vi "Cursor-Controlled Subarray.vi"(0 "cursor graph":refnum<vi>, 1 "X":dbl[](array[numeric]), 2 "Y":dbl[](array[numeric])) -> (3 "X subset":dbl[](array[numeric]), 4 "Y subset":dbl[](array[numeric]), 5 "cursor avg":dbl, 6 "cursor diff":dbl)   [LabVIEW 2015]
doc: "Allows the cursors on an XY-graph to select a subarray of that XY-graph. Also returns the difference between the two cursor positions and their average."
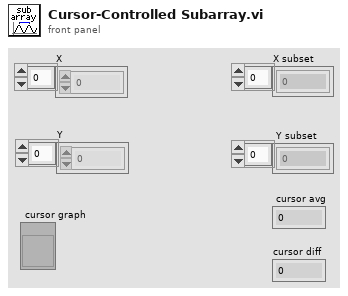
[diagram p1: front panel]
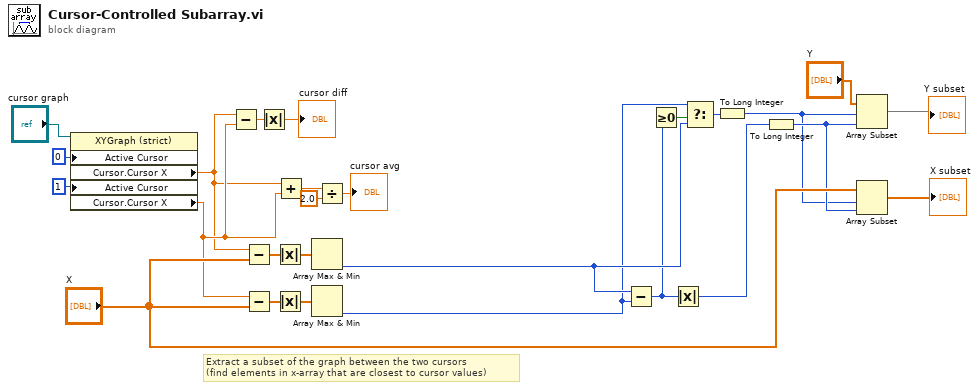
[diagram p0: block diagram]
diagram:
  # "Extract a subset of the graph between the two cursors\n(find elements in x-array that are closest to cursor values)"
  n1 = property on="Property Node" class="XYGraph (strict)"(reference="cursor graph", "Active Cursor"=u32 0, "Active Cursor"=u32 1) -> ("Cursor.Cursor X"=w19:dbl, "Cursor.Cursor X"=w20:dbl)  [unwired: 1 in, 2 out]
  n2 = Subtract(x=w19, y=w20) -> (x-y=w21:dbl)
  n3 = Subtract(x=w19, y="X") -> (x-y=w6:dbl[])
  n4 = Subtract(x=w20, y="X") -> (x-y=w4:dbl[])
  n5 = Absolute Value(x=w21) -> (abs(x)=→"cursor diff":dbl)
  n6 = Absolute Value(x=w6) -> (abs(x)=w7:dbl[])
  n7 = Absolute Value(x=w4) -> (abs(x)=w5:dbl[])
  n8 = Add(x=w19, y=w20) -> (x+y=w16:dbl)
  n9 = Array Max & Min(array=w7) -> (min index (indices)=w15:i32)  [unwired: 3 out]
  n10 = Array Max & Min(array=w5) -> (min index (indices)=w14:i32)  [unwired: 3 out]
  n11 = Divide(x=w16, y=2.0) -> (x/y=→"cursor avg":dbl)
  n12 = Subtract(x=w15, y=w14) -> (x-y=w10:i32)
  n13 = Greater Or Equal To 0?(x=w10) -> (x >= 0?=w11:bool)
  n14 = Absolute Value(x=w10) -> (abs(x)=w8:i32)
  n15 = Select(t=w14, s=w11, f=w15) -> (s? t:f=w9:i32)
  n16 = To Long Integer(number=w9) -> (32bit integer=w12:i32)
  n17 = To Long Integer(number=w8) -> (32bit integer=w13:i32)
  n18 = Array Subset ("new y-arr")(array="Y", index=w12, length=w13) -> (→"Y subset":dbl[])
  n19 = Array Subset ("new x-arr")(array="X", index=w12, length=w13) -> (→"X subset":dbl[])
